vi "HexStringToAsciiString.vi"(1 "输入Hex字符串":string) -> (0 "输出Ascii":string)   [LabVIEW 2020]
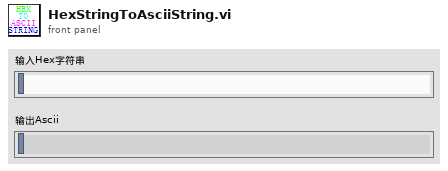
[diagram p1: front panel]
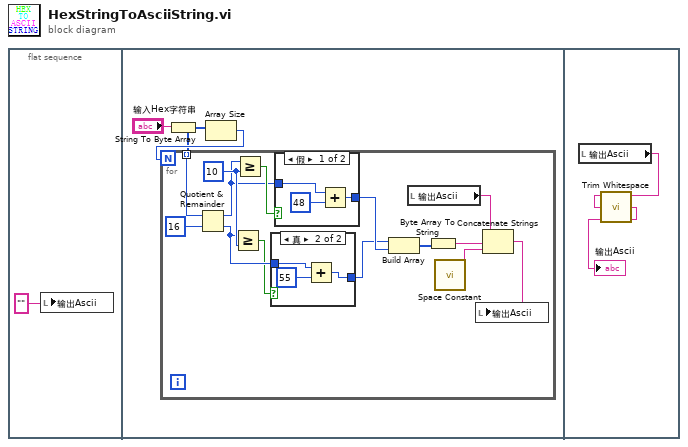
[diagram p0: block diagram]
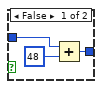
[diagram p2: hidden frame]
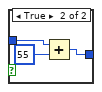
[diagram p3: hidden frame]
diagram:
  n1 = flat-sequence {
    frame #0 {
      n2 = local write "输出Ascii"("") -> ()
    }
    frame #1 {
      n3 = String To Byte Array(string="输入Hex字符串") -> (unsigned byte array=w2:u8[])
      n4 = Array Size(array=w2) -> (size(s)=w3:i32)
      n5 = for {
        N: w3 -> [_]
        tunnel: w2 -> [w18] mode=indexing
        w15 = u8 10 ("y")
        n6 = Quotient & Remainder(x=w18, y=u8 16) -> (x-y*floor(x/y)=w14:u8, floor(x/y)=w13:u8)
        n7 = Greater Or Equal?(x=w13, y=w15) -> (x >= y?=w12:bool)
        n8 = Greater Or Equal?(x=w14, y=w15) -> (x >= y?=w16:bool)
        n9 = case shown="真" w12 {
          tunnel: w13 -> [w20 w24]
          tunnel: [w19 w22] -> w10
          frame False {
            n10 = Add(x=w20, y=u8 48) -> (x+y=w19:u8)
          }
          frame True {
            n11 = Add(x=w24, y=u8 55) -> (x+y=w22:u8)
          }
        }
        n12 = case shown="假" w16 {
          tunnel: w14 -> [w26 w30]
          tunnel: [w25 w28] -> w11
          frame False {
            n13 = Add(x=w26, y=u8 48) -> (x+y=w25:u8)
          }
          frame True {
            n14 = Add(x=w30, y=u8 55) -> (x+y=w28:u8)
          }
        }
        n15 = Build Array(w10, w11) -> (w9:u8[])
        n16 = local read "输出Ascii"() -> (w7:string)
        n17 = Byte Array To String(unsigned byte array=w9) -> (string=w8:string)
        n18 = call <vilib>:"Space Constant.vi"() -> ("String"=w6:string)
        n19 = Concatenate Strings(w7, w8, w6) -> (w5:string)
        n20 = local write "输出Ascii"(w5) -> ()
      }
    }
    frame #2 {
      n21 = local read "输出Ascii"() -> (w32:string)
      n22 = call <vilib>:"Trim Whitespace.vi"("string"=w32) -> ("trimmed string"=→"输出Ascii":string)  [unwired: 1 in]
    }
  }
